vi "monochromatorDisconnect.vi"(8 "error in":errorcluster, 11 "monochromator":refnum<k24>) -> (0 "error out":errorcluster)   [LabVIEW 2009]
doc: "This VI sends disconnect request to .net assembly"
uses:
  C:/Users/anderson.chen/Desktop/Software Development/Cornerstone Series API (LV9)/Cornerstone DLL/Cornerstone.dll
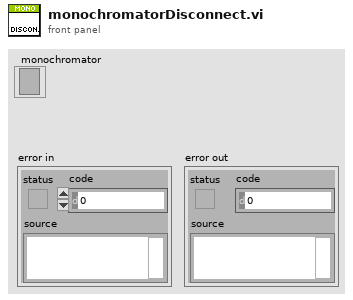
[diagram p1: front panel]
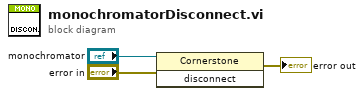
[diagram p0: block diagram]
diagram:
  n1 = invoke class="Cornerstone" method="disconnect"(reference="monochromator", error in="error in") -> (error out=→"error out":errorcluster)  [unwired: 1 in, 2 out]
